vi "Camera.CaptureImage.vi"(8 "error in (no error)":errorcluster, 11 "Camera.Simulated":refnum<class "Camera.IMAQdx.lvclass">) -> (0 "error out":errorcluster, 2 "buffer":i32, 3 "Camera.Simulated out":refnum<class "Camera.IMAQdx.lvclass">)   [LabVIEW 2020, in "Camera.IMAQdx.lvclass"]
doc: "---------------------------------------------------------------\nJKI State Machine Objects™\nhttp://jki.net/state-machine-objects/\nCopyright (C) 2005-2015, JKI <info@jki.net>\nALL RIGHTS RESERVEDJKI State Machine Objects (SMO) 1.0.0.5\nJKI - JKI\nCopyright (c) 2016, JKI"
uses:
  Camera.IMAQdx.lvclass
  Camera.IMAQdx.lvclass/Camera.IMAQdx.ctl
  Camera/Camera.lvclass
  <vilib>/vision/driver/NI_Vision_Acquisition_Software.lvlib
panel:
  # "For instructions on how to use the JKI State Machine Objects, examples and video tutorials, visit:\nhttp://jki.net/state-machine-objects/\n\nJKI State Machine Objects™\nhttp://jki.net/state-machine-objects/\nCopyright (C) 2005-2015, JKI <info@jki.net>\nALL RIGHTS RESERVED"
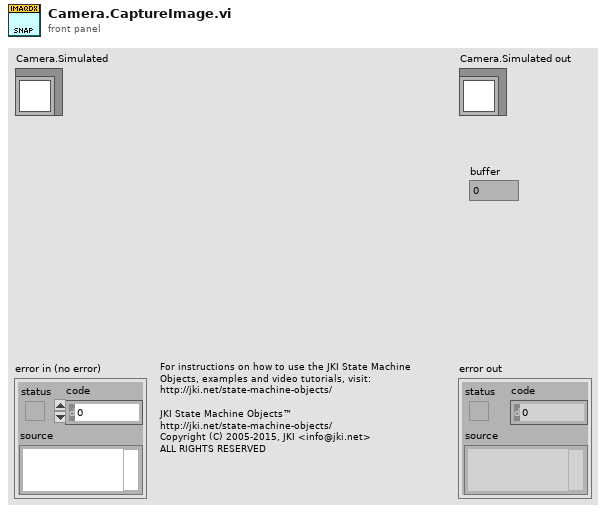
[diagram p1: front panel]
types:
  T1 = typedef "IMAQ Image.ctl" = refnum<image>
  T2 = typedef "IMAQdx.ctl" = refnum<k21>
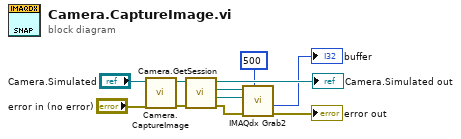
[diagram p0: block diagram]
diagram:
  n1 = call-parent "Camera.CaptureImage.vi"("error in (no error)"="error in (no error)", "Camera"="Camera.Simulated") -> ("error out"=w8:errorcluster, "Camera out"=w10:refnum<class "Camera.IMAQdx.lvclass">)  [unwired: 7 in, 1 out]
  n2 = call "Camera.GetSession.vi"("error in (no error)"=w8, "Camera.Simulated"=w10) -> ("error out"=w4:errorcluster, "Image"=w3:T1, "Session"=w1:T2, "Camera.Simulated"=→"Camera.Simulated out":refnum<class "Camera.IMAQdx.lvclass">)  [unwired: 6 in]
  n3 = call <vilib>:"IMAQdx Grab2.vi"("Timeout (ms)"=500, "error in"=w4, "Image In"=w3, "Session In"=w1) -> ("error out"=→"error out":errorcluster, "Buffer Number Out"=→"buffer":u32)  [unwired: 4 in, 2 out]
